vi "_Set Sibling.vi"(8 "error in (no error)":errorcluster, 10 "Sibling":refnum<data-value>, 11 "NodeRef In":refnum<data-value>) -> (0 "error out":errorcluster, 3 "NodeRef":refnum<data-value>)   [LabVIEW 2020, in "PicoG-ParserLexer.lvlib" / "Node.lvclass"]
doc: "Provides no protection for tree integrity. Can be used to clear sibling reference."
uses:
  Node.lvclass
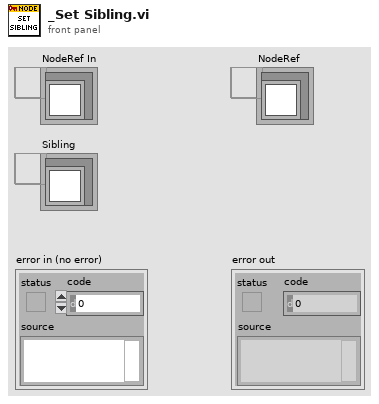
[diagram p1: front panel]
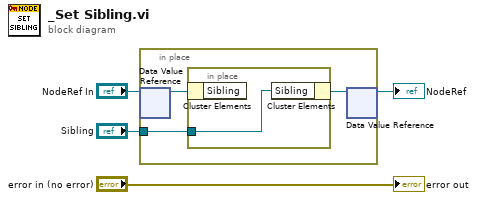
[diagram p0: block diagram]
diagram:
  n1 = in-place {
    in-place-border: "Sibling" -> [w6]
    n2 = in-place-dvr #1("NodeRef In") -> (w7:refnum<class "Node.lvclass">)  [unwired: 1 out]
    n3 = in-place {
      in-place-border: w6 -> [w8]
      n4 = in-place-cluster #2(w7) -> ()  [unwired: 1 out]
      n5 = in-place-cluster #2("Sibling"=w8) -> (w5:refnum<class "Node.lvclass">)
    }
    n6 = in-place-dvr #1(w5) -> (→"NodeRef":refnum<data-value>)  [unwired: 1 out]
  }
  "error out" <- "error in (no error)"
